vi "DIFF_DRIVE_BEGIN.vi"(8 "error in":errorcluster) -> (0 "error out":errorcluster)   [LabVIEW 2023]
uses:
  <vilib>/Rock Robotics/WPI/ThirdParty/Phoenix-LabVIEW/Motor Controller/Controls/CTRE_Phoenix_MotorControl_TalonFXInvertType.ctl
  <vilib>/Rock Robotics/WPI/ThirdParty/Phoenix-LabVIEW/Motor Controller/Controls/CTRE_Phoenix_MotorControl_FeedbackDevice.ctl
  <vilib>/Rock Robotics/WPI/ThirdParty/Phoenix-LabVIEW/Motor Controller/Controls/CTRE_Phoenix_MotorControl_NeutralMode.ctl
  <vilib>/Rock Robotics/SystemInterfaces/NetworkCommunication/NetComm_UsageReport_report.vi
  <vilib>/Rock Robotics/WPI/ThirdParty/JAS_Junk/TrajLib/Globals/Util_LibraryGlobals.vi
  <vilib>/Rock Robotics/WPI/ThirdParty/JAS_Junk/TrajLib/Trajectory_Library.lvlib
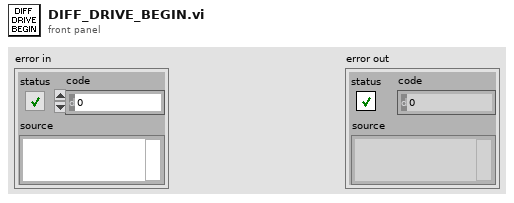
[diagram p1: front panel]
types:
  T1 = typedef "CTRE_Phoenix_MotorControl_TalonFXInvertType.ctl" = enum16{"Counter-Clockwise", "Clockwise"}
  T2 = typedef "CTRE_Phoenix_MotorControl_NeutralMode.ctl" = enum8{"EEPROMSetting", "Override to Coast", "Override to Brake"}
  T3 = typedef "CTRE_Phoenix_MotorControl_FeedbackDevice.ctl" = i8
  T4 = typedef "WPI_MotorControlDeviceRef.ctl" = cluster{"DeviceStatus":errorcluster, "Type":T5, "PWM":cluster{"PWM Channel":T6, "DeadBand":T7}, "CAN":cluster{"Device Number":u8, "SetOutput VI Ref":variant, "GetOutput VI Ref":variant, "Enable VI Ref":variant, "Disable VI Ref":variant, "Data":variant}, "Invert":bool, "DIO PWM":cluster{"PWM \"Enable\" Channel":T6, "DIOChannel":T8, "PWM Rate":dbl}}
  T5 = typedef "WPI_MotorControlType.ctl" = enum16{"PWM", "CAN", "DIO PWM"}
  T6 = typedef "FPGA_DIOPWMChannel.ctl" = enum8{"PWM 0", "PWM 1", "PWM 2", "PWM 3", "PWM 4", "PWM 5", "PWM 6", "PWM 7", "PWM 8", "PWM 9", "PWM MXP 0", "PWM MXP 1", "PWM MXP 2", "PWM MXP 3", "PWM MXP 4", "PWM MXP 5", "PWM MXP 6", "PWM MXP 7", "PWM MXP 8", "PWM MXP 9", "Invalid"}
  T7 = typedef "WPI_PWMDeadband.ctl" = cluster{"Name":string, "maxPositivePwm":i32, "minPositivePwm":i32, "centerPwm":i32, "maxNegativePwm":i32, "minNegativePwm":i32, "angularRange":u16}
  T8 = typedef "FPGA_DIOChannel.ctl" = enum8{"DIO 0", "DIO 1", "DIO 2", "DIO 3", "DIO 4", "DIO 5", "DIO 6", "DIO 7", "DIO 8", "DIO 9", "DIO MXP 0", "DIO MXP 1", "DIO MXP 2", "DIO MXP 3", "DIO MXP 4", "DIO MXP 5", "DIO MXP 6", "DIO MXP 7", "DIO MXP 8", "DIO MXP 9", "DIO MXP 10", "DIO MXP 11", "DIO MXP 12", "DIO MXP 13", "DIO MXP 14", "DIO MXP 15", "SPI Port CS1", "SPI Port CS2", "SPI Port CS3", "SPI Port MISO", "SPI Port MOSI", "Invalid"}
  T9 = typedef "Trajectory_Library.lvlib/DIFF_DRIVE_KINEMATICS.ctl" = cluster{"TrackWidth_Meters":dbl}
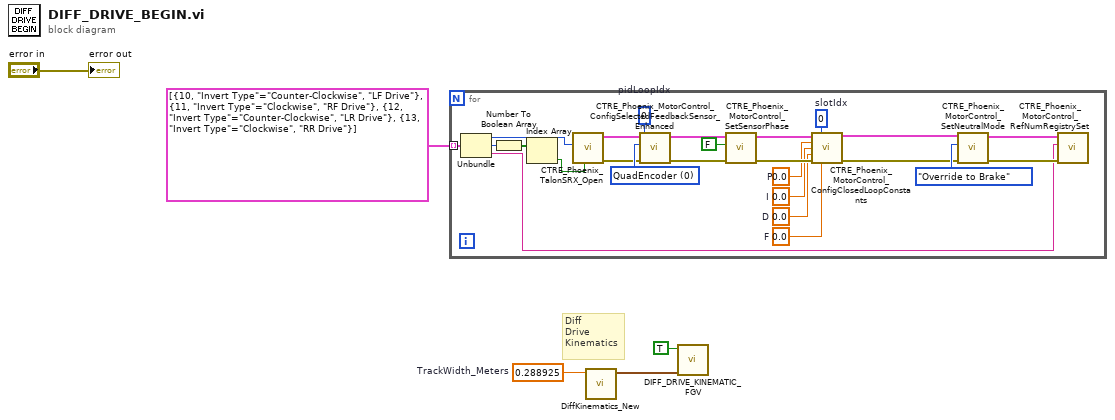
[diagram p0: block diagram]
diagram:
  w3 = 0.288925  # TrackWidth_Meters
  # "Diff\nDrive\nKinematics"
  n1 = for {
    tunnel: cluster{i32, "Invert Type":T1, string}[] [{10, "Invert Type"=enum."Counter-Clockwise", "LF Drive"}, {11, "Invert Type"=enum."Clockwise", "RF Drive"}, {12, "Invert Type"=enum."Counter-Clockwise", "LR Drive"}, {13, "Invert Type"=enum."Clockwise", "RR Drive"}] ("Array") -> [w30] mode=indexing
    w6 = 0  # slotIdx
    w9 = 0.0  # F
    w10 = 0.0  # D
    w11 = 0.0  # I
    w12 = 0.0  # P
    w18 = 0  # pidLoopIdx
    w21 = T3 0 items=["QuadEncoder"=0, "Analog"=2, "Tachometer"=4, "Pulse Width Encoded Position"=8, "Sensor Sum (S0 + S1)"=9, "Sensor Difference (D0 - D1)"=10, "Remote Source 0"=11, "Remote Source 1"=12, "Software Emulated"=15] ("Feedback Device")
    n2 = Unbundle(w30) -> (w23:i32, "Invert Type"=w28:T1, w24:string)
    n3 = Number To Boolean Array(number=w28) -> (Boolean array=w29:bool[])
    n4 = Index Array(array=w29) -> (element=w22:bool)  [unwired: 1 in]
    n5 = call <vilib>:"CTRE_Phoenix_TalonSRX_Open.vi"("Invert"=w22, "Device Number"=w23) -> ("error out"=w19:errorcluster, "PhoenixMotorControlDevRef"=w20:T4)  [unwired: 8 in]
    n6 = call <vilib>:"CTRE_Phoenix_MotorControl_ConfigSelectedFeedbackSensor_Enhanced.vi"("error in (no error)"=w19, "pidLoopIdx"=w18, "Feedback Device"=w21, "PhoenixMotorControlDevRef"=w20) -> ("error out"=w15:errorcluster, "PhoenixMotorControlDevRef"=w16:T4)  [unwired: 6 in]
    n7 = call <vilib>:"CTRE_Phoenix_MotorControl_SetSensorPhase.vi"("error in (no error)"=w15, "PhaseSensor"=FALSE, "PhoenixMotorControlDevRef"=w16) -> ("error out"=w13:errorcluster, "PhoenixMotorControlDevRef"=w14:T4)  [unwired: 7 in]
    n8 = call <vilib>:"CTRE_Phoenix_MotorControl_ConfigClosedLoopConstants.vi"("PhoenixMotorControlDevRef"=w14, "slotIdx"=w6, "P"=w12, "I"=w11, "D"=w10, "error in (no error)"=w13, "F"=w9) -> ("PhoenixMotorControlDevRef"=w8:T4, "error out"=w7:errorcluster)  [unwired: 7 in]
    n9 = call <vilib>:"CTRE_Phoenix_MotorControl_SetNeutralMode.vi"("error in (no error)"=w7, "Motor Control Neutral Mode"=CTRE_Phoenix_MotorControl_NeutralMode."Override to Brake", "PhoenixMotorControlDevRef"=w8) -> ("error out"=w26:errorcluster, "PhoenixMotorControlDevRef"=w27:T4)  [unwired: 7 in]
    n10 = call <vilib>:"CTRE_Phoenix_MotorControl_RefNumRegistrySet.vi"("error in (no error)"=w26, "refnum name"=w24, "PhoenixMotorControlDevRef"=w27) -> ()  [unwired: 7 in, 2 out]
  }
  n11 = call <vilib>:"DiffKinematics_New.vi"("TrackWidth_Meters"=w3) -> ("DIFF_DRIVE_KINEMATICS"=w2:T9)  [unwired: 10 in]
  n12 = call "DIFF_DRIVE_KINEMATIC_FGV.vi"("in DIFF_DRIVE_KINEMATICS"=w2, "Write"=TRUE) -> ()  [unwired: 9 in, 1 out]
  "error out" <- "error in"
